vi "LHPulse-10-06-17.vi"(1 "LHPulse(us)":T1, 2 "LHHeizen2?":T2, 3 "LHHeizen1?":T2) -> ()   [LabVIEW 2017]
uses:
  <vilib>/rvi/eio/common/nirviEmuTemplateMethod_errors.vi
  <vilib>/eio/EIONode/EIONode.xnode
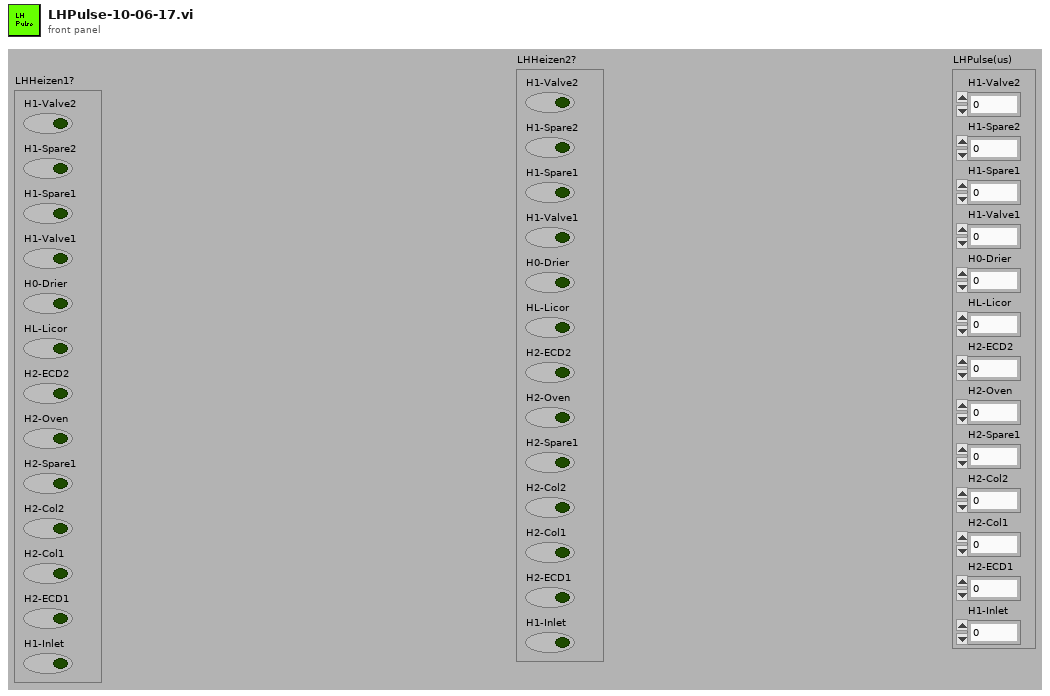
[diagram p1: front panel]
types:
  T1 = cluster{"H1-Valve2":u32, "H1-Spare2":u32, "H1-Spare1":u32, "H1-Valve1":u32, "H0-Drier":u32, "HL-Licor":u32, "H2-ECD2":u32, "H2-Oven":u32, "H2-Spare1":u32, "H2-Col2":u32, "H2-Col1":u32, "H2-ECD1":u32, "H1-Inlet":u32}
  T2 = cluster{"H1-Valve2":bool, "H1-Spare2":bool, "H1-Spare1":bool, "H1-Valve1":bool, "H0-Drier":bool, "HL-Licor":bool, "H2-ECD2":bool, "H2-Oven":bool, "H2-Spare1":bool, "H2-Col2":bool, "H2-Col1":bool, "H2-ECD1":bool, "H1-Inlet":bool}
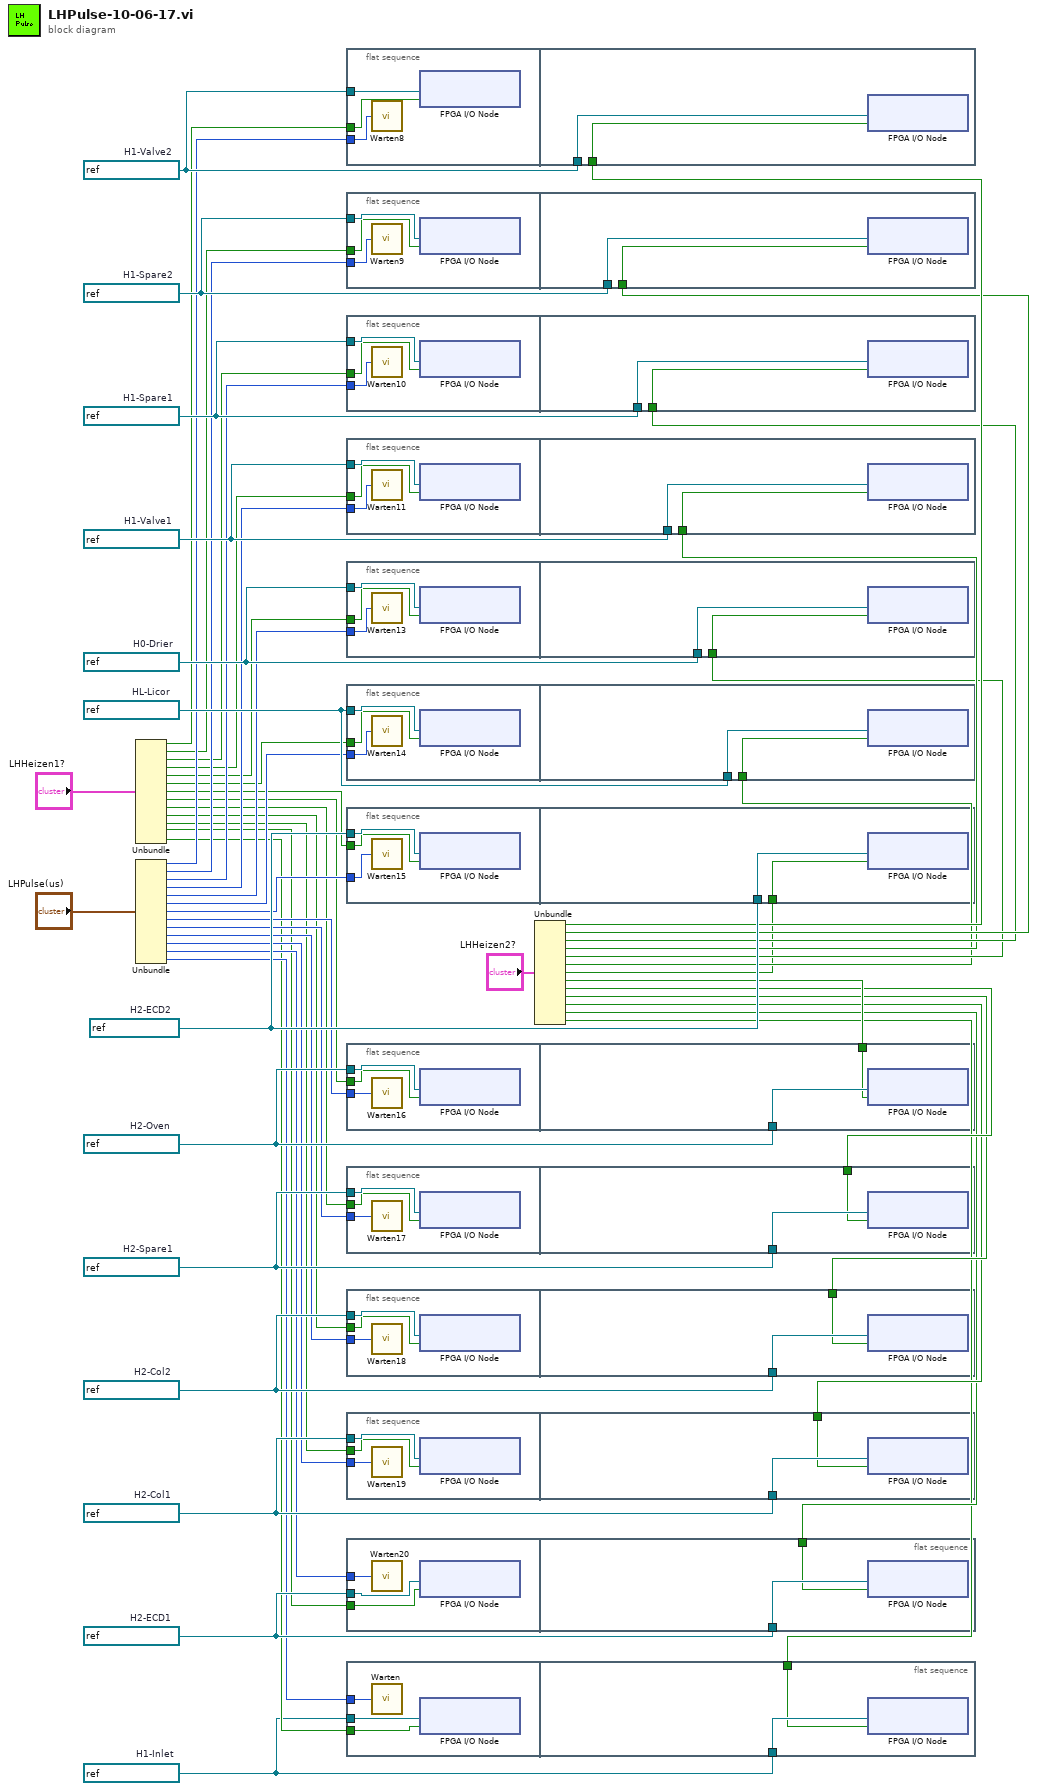
[diagram p0: block diagram]
diagram:
  w1 = refnum<k21> "Mod5/DIO14"  # H1-Inlet
  w44 = refnum<k21> "Mod5/DIO20"  # H2-ECD1
  w45 = refnum<k21> "Mod5/DIO19"  # H2-Col1
  w46 = refnum<k21> "Mod5/DIO18"  # H2-Col2
  w47 = refnum<k21> "Mod5/DIO17"  # H2-Spare1
  w48 = refnum<k21> "Mod5/DIO16"  # H2-Oven
  w49 = refnum<k21> "Mod5/DIO1"  # H2-ECD2
  w50 = refnum<k21> "Mod5/DIO27"  # HL-Licor
  w51 = refnum<k21> "Mod5/DIO31"  # H0-Drier
  w52 = refnum<k21> "Mod6/DIO27"  # H1-Valve1
  w53 = refnum<k21> "Mod6/DIO26"  # H1-Spare1
  w54 = refnum<k21> "Mod6/DIO25"  # H1-Spare2
  w55 = refnum<k21> "Mod6/DIO24"  # H1-Valve2
  n1 = Unbundle("LHHeizen1?") -> ("H1-Valve2"=w31:bool, "H1-Spare2"=w30:bool, "H1-Spare1"=w29:bool, "H1-Valve1"=w28:bool, "H0-Drier"=w27:bool, "HL-Licor"=w26:bool, "H2-ECD2"=w25:bool, "H2-Oven"=w24:bool, "H2-Spare1"=w23:bool, "H2-Col2"=w22:bool, "H2-Col1"=w21:bool, "H2-ECD1"=w20:bool, "H1-Inlet"=w3:bool)
  n2 = Unbundle("LHPulse(us)") -> ("H1-Valve2"=w43:u32, "H1-Spare2"=w42:u32, "H1-Spare1"=w41:u32, "H1-Valve1"=w40:u32, "H0-Drier"=w39:u32, "HL-Licor"=w38:u32, "H2-ECD2"=w37:u32, "H2-Oven"=w36:u32, "H2-Spare1"=w35:u32, "H2-Col2"=w34:u32, "H2-Col1"=w33:u32, "H2-ECD1"=w32:u32, "H1-Inlet"=w4:u32)
  n3 = flat-sequence {
    tunnel: w55 -> [w58]
    tunnel: w31 -> [w57]
    tunnel: w43 -> [w56]
    tunnel: w55 -> [w60]
    tunnel: w19 -> [w59]
    frame #0 {
      n4 = call "Warten8"("Count(uSec)"=w56) -> ()  [unwired: 1 out]
      n5 = xnode "FPGA I/O Node"("I/O-Objekt"=w57, "FPGA-I/O (Eingang)"=w58) -> ()  [unwired: 1 out]
    }
    frame #1 {
      n6 = xnode "FPGA I/O Node"("I/O-Objekt"=w59, "FPGA-I/O (Eingang)"=w60) -> ()  [unwired: 1 out]
    }
  }
  n7 = flat-sequence {
    tunnel: w54 -> [w63]
    tunnel: w30 -> [w62]
    tunnel: w42 -> [w61]
    tunnel: w54 -> [w65]
    tunnel: w18 -> [w64]
    frame #0 {
      n8 = call "Warten9"("Count(uSec)"=w61) -> ()  [unwired: 1 out]
      n9 = xnode "FPGA I/O Node"("I/O-Objekt"=w62, "FPGA-I/O (Eingang)"=w63) -> ()  [unwired: 1 out]
    }
    frame #1 {
      n10 = xnode "FPGA I/O Node"("I/O-Objekt"=w64, "FPGA-I/O (Eingang)"=w65) -> ()  [unwired: 1 out]
    }
  }
  n11 = flat-sequence {
    tunnel: w53 -> [w68]
    tunnel: w29 -> [w67]
    tunnel: w41 -> [w66]
    tunnel: w53 -> [w70]
    tunnel: w17 -> [w69]
    frame #0 {
      n12 = call "Warten10"("Count(uSec)"=w66) -> ()  [unwired: 1 out]
      n13 = xnode "FPGA I/O Node"("I/O-Objekt"=w67, "FPGA-I/O (Eingang)"=w68) -> ()  [unwired: 1 out]
    }
    frame #1 {
      n14 = xnode "FPGA I/O Node"("I/O-Objekt"=w69, "FPGA-I/O (Eingang)"=w70) -> ()  [unwired: 1 out]
    }
  }
  n15 = flat-sequence {
    tunnel: w52 -> [w73]
    tunnel: w28 -> [w72]
    tunnel: w40 -> [w71]
    tunnel: w52 -> [w75]
    tunnel: w16 -> [w74]
    frame #0 {
      n16 = call "Warten11"("Count(uSec)"=w71) -> ()  [unwired: 1 out]
      n17 = xnode "FPGA I/O Node"("I/O-Objekt"=w72, "FPGA-I/O (Eingang)"=w73) -> ()  [unwired: 1 out]
    }
    frame #1 {
      n18 = xnode "FPGA I/O Node"("I/O-Objekt"=w74, "FPGA-I/O (Eingang)"=w75) -> ()  [unwired: 1 out]
    }
  }
  n19 = flat-sequence {
    tunnel: w51 -> [w78]
    tunnel: w27 -> [w77]
    tunnel: w39 -> [w76]
    tunnel: w51 -> [w80]
    tunnel: w15 -> [w79]
    frame #0 {
      n20 = call "Warten13"("Count(uSec)"=w76) -> ()  [unwired: 1 out]
      n21 = xnode "FPGA I/O Node"("I/O-Objekt"=w77, "FPGA-I/O (Eingang)"=w78) -> ()  [unwired: 1 out]
    }
    frame #1 {
      n22 = xnode "FPGA I/O Node"("I/O-Objekt"=w79, "FPGA-I/O (Eingang)"=w80) -> ()  [unwired: 1 out]
    }
  }
  n23 = flat-sequence {
    tunnel: w50 -> [w83]
    tunnel: w26 -> [w82]
    tunnel: w38 -> [w81]
    tunnel: w50 -> [w85]
    tunnel: w14 -> [w84]
    frame #0 {
      n24 = call "Warten14"("Count(uSec)"=w81) -> ()  [unwired: 1 out]
      n25 = xnode "FPGA I/O Node"("I/O-Objekt"=w82, "FPGA-I/O (Eingang)"=w83) -> ()  [unwired: 1 out]
    }
    frame #1 {
      n26 = xnode "FPGA I/O Node"("I/O-Objekt"=w84, "FPGA-I/O (Eingang)"=w85) -> ()  [unwired: 1 out]
    }
  }
  n27 = flat-sequence {
    tunnel: w49 -> [w88]
    tunnel: w25 -> [w87]
    tunnel: w37 -> [w86]
    tunnel: w49 -> [w90]
    tunnel: w13 -> [w89]
    frame #0 {
      n28 = call "Warten15"("Count(uSec)"=w86) -> ()  [unwired: 1 out]
      n29 = xnode "FPGA I/O Node"("I/O-Objekt"=w87, "FPGA-I/O (Eingang)"=w88) -> ()  [unwired: 1 out]
    }
    frame #1 {
      n30 = xnode "FPGA I/O Node"("I/O-Objekt"=w89, "FPGA-I/O (Eingang)"=w90) -> ()  [unwired: 1 out]
    }
  }
  n31 = flat-sequence {
    tunnel: w48 -> [w93]
    tunnel: w24 -> [w92]
    tunnel: w36 -> [w91]
    tunnel: w48 -> [w95]
    tunnel: w12 -> [w94]
    frame #0 {
      n32 = call "Warten16"("Count(uSec)"=w91) -> ()  [unwired: 1 out]
      n33 = xnode "FPGA I/O Node"("I/O-Objekt"=w92, "FPGA-I/O (Eingang)"=w93) -> ()  [unwired: 1 out]
    }
    frame #1 {
      n34 = xnode "FPGA I/O Node"("I/O-Objekt"=w94, "FPGA-I/O (Eingang)"=w95) -> ()  [unwired: 1 out]
    }
  }
  n35 = flat-sequence {
    tunnel: w47 -> [w98]
    tunnel: w23 -> [w97]
    tunnel: w35 -> [w96]
    tunnel: w47 -> [w100]
    tunnel: w11 -> [w99]
    frame #0 {
      n36 = call "Warten17"("Count(uSec)"=w96) -> ()  [unwired: 1 out]
      n37 = xnode "FPGA I/O Node"("I/O-Objekt"=w97, "FPGA-I/O (Eingang)"=w98) -> ()  [unwired: 1 out]
    }
    frame #1 {
      n38 = xnode "FPGA I/O Node"("I/O-Objekt"=w99, "FPGA-I/O (Eingang)"=w100) -> ()  [unwired: 1 out]
    }
  }
  n39 = flat-sequence {
    tunnel: w46 -> [w103]
    tunnel: w22 -> [w102]
    tunnel: w34 -> [w101]
    tunnel: w46 -> [w105]
    tunnel: w10 -> [w104]
    frame #0 {
      n40 = call "Warten18"("Count(uSec)"=w101) -> ()  [unwired: 1 out]
      n41 = xnode "FPGA I/O Node"("I/O-Objekt"=w102, "FPGA-I/O (Eingang)"=w103) -> ()  [unwired: 1 out]
    }
    frame #1 {
      n42 = xnode "FPGA I/O Node"("I/O-Objekt"=w104, "FPGA-I/O (Eingang)"=w105) -> ()  [unwired: 1 out]
    }
  }
  n43 = flat-sequence {
    tunnel: w45 -> [w108]
    tunnel: w21 -> [w107]
    tunnel: w33 -> [w106]
    tunnel: w45 -> [w110]
    tunnel: w9 -> [w109]
    frame #0 {
      n44 = call "Warten19"("Count(uSec)"=w106) -> ()  [unwired: 1 out]
      n45 = xnode "FPGA I/O Node"("I/O-Objekt"=w107, "FPGA-I/O (Eingang)"=w108) -> ()  [unwired: 1 out]
    }
    frame #1 {
      n46 = xnode "FPGA I/O Node"("I/O-Objekt"=w109, "FPGA-I/O (Eingang)"=w110) -> ()  [unwired: 1 out]
    }
  }
  n47 = flat-sequence {
    tunnel: w44 -> [w113]
    tunnel: w20 -> [w112]
    tunnel: w32 -> [w111]
    tunnel: w44 -> [w115]
    tunnel: w8 -> [w114]
    frame #0 {
      n48 = call "Warten20"("Count(uSec)"=w111) -> ()  [unwired: 1 out]
      n49 = xnode "FPGA I/O Node"("I/O-Objekt"=w112, "FPGA-I/O (Eingang)"=w113) -> ()  [unwired: 1 out]
    }
    frame #1 {
      n50 = xnode "FPGA I/O Node"("I/O-Objekt"=w114, "FPGA-I/O (Eingang)"=w115) -> ()  [unwired: 1 out]
    }
  }
  n51 = flat-sequence {
    tunnel: w1 -> [w118]
    tunnel: w3 -> [w117]
    tunnel: w4 -> [w116]
    tunnel: w1 -> [w120]
    tunnel: w2 -> [w119]
    frame #0 {
      n52 = call "Warten"("Count(uSec)"=w116) -> ()  [unwired: 1 out]
      n53 = xnode "FPGA I/O Node"("I/O-Objekt"=w117, "FPGA-I/O (Eingang)"=w118) -> ()  [unwired: 1 out]
    }
    frame #1 {
      n54 = xnode "FPGA I/O Node"("I/O-Objekt"=w119, "FPGA-I/O (Eingang)"=w120) -> ()  [unwired: 1 out]
    }
  }
  n55 = Unbundle("LHHeizen2?") -> ("H1-Valve2"=w19:bool, "H1-Spare2"=w18:bool, "H1-Spare1"=w17:bool, "H1-Valve1"=w16:bool, "H0-Drier"=w15:bool, "HL-Licor"=w14:bool, "H2-ECD2"=w13:bool, "H2-Oven"=w12:bool, "H2-Spare1"=w11:bool, "H2-Col2"=w10:bool, "H2-Col1"=w9:bool, "H2-ECD1"=w8:bool, "H1-Inlet"=w2:bool)
